vi "Run-TimePosition.GetPosition.vi"(8 "error in (no error)":errorcluster, 11 "WindowFrame in":refnum<class "WindowFrame.lvclass">) -> (0 "error out":errorcluster, 2 "GetPosition":T1, 3 "WindowFrame out":refnum<class "WindowFrame.lvclass">)   [LabVIEW 2021, in "WindowFrame.lvlib" / "WindowFrame.lvclass"]
uses:
  WindowFrame.lvclass
  FrontPanel.Run-TimePosition.GetPosition.ctl
  Action.ctl
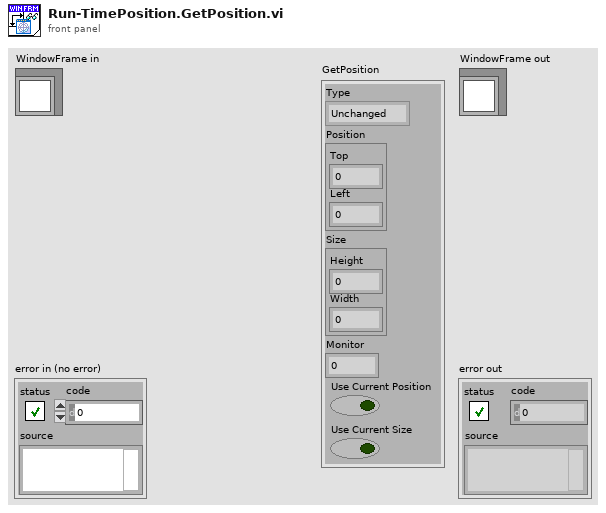
[diagram p1: front panel]
types:
  T1 = typedef "WindowFrame.lvlib/WindowFrame.lvclass/FrontPanel.Run-TimePosition.GetPosition.ctl" = cluster{"Type":enum32{"Unchanged", "Centered", "Maximized", "Minimized", "Custom"}, "Position":cluster{"Top":i16, "Left":i16}, "Size":cluster{"Height":i16, "Width":i16}, "Monitor":i16, "Use Current Position":bool, "Use Current Size":bool}
  T2 = typedef "WindowFrame.lvlib/WindowFrame.lvclass/Action.ctl" = enum16{"Set Allow Runtime PopUp", "Set Behavior", "Set Closable", "Set Custom Title", "Set Highlight Return Button", "Set Is Frontmost", "Set Minimizable", "Set Minimum Size", "Set Monitor", "Set Resizable", "Set Panel Bounds", "Set Run VI Transparently", "Set Show Menu Bar", "Set State", "Set Title", "Set Title Bar Colors", "Set Title Bar Visible", "Set Transparancy", "Set Window Bounds", "Get Allow Runtime PopUp", "Get Behavior", "Get Closable", "Get Custom Title", "Get Highlight Return Button", "Get Is Frontmost", "Get Minimizable", "Get Minimum Size", "Get Monitor", "Get Panel Bounds", "Get Resizable", "Get Run VI Transparently", "Get Show Menu Bar", "Get State", "Get Title", "Get Title Bar Colors", "Get Title Bar Visible", "Get Transparancy", "Get Window Bounds", "--", "Center", "Close", "Open", "Run-Time Position:Centered", "Run-Time Position:Custom", "Run-Time Position:Get Position", "Run-Time Position:Maximized", "Run-Time Position:Minimized", "Run-Time Position:Unchanged", "---", "Insert VI", "Remove VI", "Insert VI Index", "Remove VI Index", "Exit"}
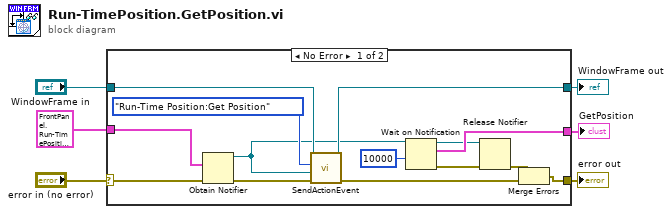
[diagram p0: block diagram]
diagram:
  n1 = case shown="No Error" "error in (no error)" {
    selector: "error in (no error)" -> [w16 w23]
    tunnel: [w11 w23] -> w5
    tunnel: [w20 w22] -> w3
    tunnel: "WindowFrame in" -> [w19 w22]
    tunnel: [w12 w21] -> w2
    tunnel: T1 {"Type"=enum."Unchanged", "Position"={"Top"=0, "Left"=0}, "Size"={"Height"=0, "Width"=0}, "Monitor"=0, "Use Current Position"=FALSE, "Use Current Size"=FALSE} ("GetPosition") -> [w14 w21]
    frame No Error {
      n2 = Obtain Notifier(notification data type=w14, error in (no error)=w16) -> (notifier out=w13:refnum<notifier>, error out=w15:errorcluster)  [unwired: 2 in, 1 out]
      n3 = call "SendActionEvent.vi"("error in (no error)"=w15, "Variant"=w13, "Action"=Action."Run-Time Position:Get Position", "WindowFrame in"=w19) -> ("error out"=w18:errorcluster, "WindowFrame out"=w20:refnum<class "WindowFrame.lvclass">)  [unwired: 6 in]
      n4 = Wait on Notification(notifier=w13, timeout in ms (-1)=10000) -> (notifier out=w7:refnum<notifier>, notification=w12:T1, error out=w10:errorcluster)  [unwired: 2 in, 1 out]
      n5 = Release Notifier(notifier=w7, error in (no error)=w10) -> (error out=w8:errorcluster)  [unwired: 1 in, 2 out]
      n6 = Merge Errors(w8, w18) -> (w11:errorcluster)
    }
    frame Error {
    }
  }
  "error out" <- w5
  "WindowFrame out" <- w3
  "GetPosition" <- w2
